vi "Wait Socket.vi"   [LabVIEW 2013, in "libssh2.lvlib"]
doc: "Wait for data on a socket in reading or writing direction as indicated by the session."
uses:
  libssh2.lvlib
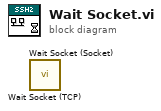
[diagram p0: block diagram]
diagram:
  n1 = call "Wait Socket (TCP).vi"() -> ()  [unwired: 11 in, 1 out]
  n2 = call "Wait Socket (Socket).vi"() -> ()  [unwired: 11 in, 1 out]
